vi "ReadFlattenImageOptions.vi"(8 "error in":errorcluster) -> (0 "error out":errorcluster, 1 "Type of Flatten":T1 items=["Image", "Image and Vision Info", "Reference to Image"], 2 "Quality":i32=750, 3 "Compression (None)":T2 items=["None", "JPEG", "PACKED BINARY"])   [LabVIEW 2020, in "OpenLvVision_Image.lvlib" / "DataAccess.lvlib"]
doc: "These options dictate how images are compressed when converted to a string using the LabVIEW \"Flatten To String\" function."
uses:
  DataAccess.lvlib
  TypeDef/FlattenCompression.ctl
  TypeDef/TypeOfFlatten.ctl
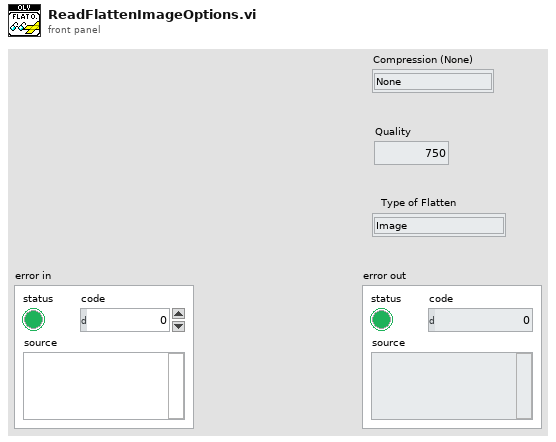
[diagram p1: front panel]
types:
  T1 = typedef "OpenLvVision_Image.lvlib/DataAccess.lvlib/TypeOfFlatten.ctl" = i32
  T2 = typedef "OpenLvVision_Image.lvlib/DataAccess.lvlib/FlattenCompression.ctl" = i32
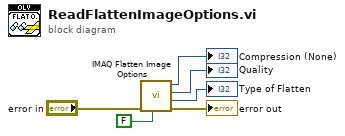
[diagram p0: block diagram]
diagram:
  n1 = call "IMAQ Flatten Image Options"("Get/Set Status? (Set)"=FALSE, "error in (no error)"="error in") -> ("error out"=→"error out":errorcluster, "Type of Flatten"=→"Type of Flatten":i32, "Quality"=→"Quality":i32, "Compression"=→"Compression (None)":i32)  [unwired: 6 in]
